vi "AUTO ERRO RBIT.vi"() -> (1 "logical AND":bool, 3 "element 2":string)   [LabVIEW 2015]
uses:
  Galobal variable_TI.vi
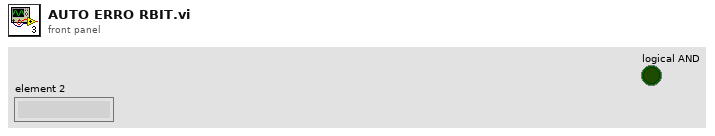
[diagram p1: front panel]
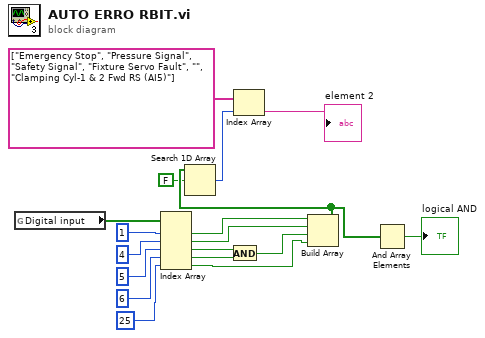
[diagram p0: block diagram]
diagram:
  n1 = global read "Galobal variable_TI.vi" "Digital input"() -> (w2:bool[])
  n2 = Index Array(array=w2, index #1=1 ("index"), index #2=4 ("index"), index #3=5 ("index"), index #4=6 ("index"), index #5=25 ("index")) -> (element #1=w9:bool, element #2=w10:bool, element #3=w11:bool, element #4=w12:bool, element #5=w16:bool)
  n3 = And(x=w11, y=w12) -> (x .and. y?=w14:bool)
  n4 = Build Array(w9, w10, w14, w16) -> (w18:bool[])
  n5 = Search 1D Array(1D array=w18, element=FALSE) -> (index of element=w8:i32)  [unwired: 1 in]
  n6 = Index Array(array=string[] ["Emergency Stop", "Pressure Signal", "Safety Signal", "Fixture Servo Fault", "", "Clamping Cyl-1 & 2 Fwd RS (AI5)"], index=w8) -> (element=→"element 2":string)
  n7 = And Array Elements(Boolean array=w18) -> (logical AND=→"logical AND":bool)
